vi "HFRR ADV v09.vi"() -> ()   [LabVIEW 2025] (continued)
            n2119 = Delete From Array(array=w2342, index=0) -> (array with subset deleted=w2264:dbl[])  [unwired: 1 in, 1 out]
            n2120 = Delete From Array(array=w2302, index=0) -> (array with subset deleted=w2260:dbl[])  [unwired: 1 in, 1 out]
            n2121 = Delete From Array(array=w2351, index=0) -> (array with subset deleted=w2265:dbl[])  [unwired: 1 in, 1 out]
            n2122 = Delete From Array(array=w2304, index=0) -> (array with subset deleted=w2261:dbl[])  [unwired: 1 in, 1 out]
            n2123 = Delete From Array(array=w2285, index=0) -> (array with subset deleted=w2257:dbl[])  [unwired: 1 in, 1 out]
            n2124 = Delete From Array(array=w2329, index=0) -> (array with subset deleted=w2315:dbl[])  [unwired: 1 in, 1 out]
            n2125 = Delete From Array(array=w2356, index=0) -> (array with subset deleted=w2317:dbl[])  [unwired: 1 in, 1 out]
            n2126 = Delete From Array(array=w2333, index=0) -> (array with subset deleted=w2263:dbl[])  [unwired: 1 in, 1 out]
            n2127 = Delete From Array(array=w2300, index=0) -> (array with subset deleted=w2259:dbl[])  [unwired: 1 in, 1 out]
            n2128 = Delete From Array(array=w2281, index=0) -> (array with subset deleted=w2255:dbl[])  [unwired: 1 in, 1 out]
            n2129 = Delete From Array(array=w2325, index=0) -> (array with subset deleted=w2313:dbl[])  [unwired: 1 in, 1 out]
            n2130 = Delete From Array(array=w2338, index=0) -> (array with subset deleted=w2318:dbl[])  [unwired: 1 in, 1 out]
            n2131 = Delete From Array(array=w2348, index=0) -> (array with subset deleted=w2231:dbl[])  [unwired: 1 in, 1 out]
            n2132 = Delete From Array(array=w2358, index=0) -> (array with subset deleted=w2233:dbl[])  [unwired: 1 in, 1 out]
            n2133 = Delete From Array(array=w2340, index=0) -> (array with subset deleted=w2229:dbl[])  [unwired: 1 in, 1 out]
            n2134 = Bundle "Bundle"(w2235, w2266) -> (w2253:cluster{dbl[], dbl[]})  [unwired: 1 in]
            n2135 = Bundle "Bundle"(w2235, w2320) -> (w2254:cluster{dbl[], dbl[]})  [unwired: 1 in]
            n2136 = Bundle "Bundle"(w2266, w2262) -> (w2268:cluster{dbl[], dbl[]})  [unwired: 1 in]
            n2137 = Bundle "Bundle"(w2231, w2230) -> (w2238:cluster{dbl[], dbl[]})  [unwired: 1 in]
            n2138 = Bundle "Bundle"(w2264, w2260) -> (w2270:cluster{dbl[], dbl[]})  [unwired: 1 in]
            n2139 = Bundle "Bundle"(w2231, w2264) -> (w2374:cluster{dbl[], dbl[]})  [unwired: 1 in]
            n2140 = Bundle "Bundle"(w2231, w2260) -> (w2298:cluster{dbl[], dbl[]})  [unwired: 1 in]
            n2141 = Bundle "Bundle"(w2231, w2319) -> (w2384:cluster{dbl[], dbl[]})  [unwired: 1 in]
            n2142 = Bundle "Bundle"(w2231, w2314) -> (w2322:cluster{dbl[], dbl[]})  [unwired: 1 in]
            n2143 = Bundle "Bundle"(w2231, w2345) -> (w2369:cluster{dbl[], dbl[]})  [unwired: 1 in]
            n2144 = Bundle "Bundle"(w2265, w2261) -> (w2269:cluster{dbl[], dbl[]})  [unwired: 1 in]
            n2145 = Bundle "Bundle"(w2233, w2232) -> (w2239:cluster{dbl[], dbl[]})  [unwired: 1 in]
            n2146 = Bundle "Bundle"(w2233, w2265) -> (w2376:cluster{dbl[], dbl[]})  [unwired: 1 in]
            n2147 = Bundle "Bundle"(w2233, w2261) -> (w2299:cluster{dbl[], dbl[]})  [unwired: 1 in]
            n2148 = Bundle "Bundle"(w2233, w2315) -> (w2323:cluster{dbl[], dbl[]})  [unwired: 1 in]
            n2149 = Bundle "Bundle"(w2233, w2317) -> (w2385:cluster{dbl[], dbl[]})  [unwired: 1 in]
            n2150 = Bundle "Bundle"(w2233, w2354) -> (w2367:cluster{dbl[], dbl[]})  [unwired: 1 in]
            n2151 = Bundle "Bundle"(w2263, w2259) -> (w2271:cluster{dbl[], dbl[]})  [unwired: 1 in]
            n2152 = Bundle "Bundle"(w2229, w2228) -> (w2237:cluster{dbl[], dbl[]})  [unwired: 1 in]
            n2153 = Bundle "Bundle"(w2229, w2263) -> (w2375:cluster{dbl[], dbl[]})  [unwired: 1 in]
            n2154 = Bundle "Bundle"(w2229, w2259) -> (w2297:cluster{dbl[], dbl[]})  [unwired: 1 in]
            n2155 = Bundle "Bundle"(w2229, w2313) -> (w2321:cluster{dbl[], dbl[]})  [unwired: 1 in]
            n2156 = Bundle "Bundle"(w2229, w2318) -> (w2383:cluster{dbl[], dbl[]})  [unwired: 1 in]
            n2157 = Bundle "Bundle"(w2229, w2336) -> (w2368:cluster{dbl[], dbl[]})  [unwired: 1 in]
            n2158 = call-poly <vilib>:"Mean.vi"("X"=w2316) -> ("mean"=→"CP1":dbl)  [unwired: 1 out]
            n2159 = call-poly <vilib>:"Mean.vi"("X"=w2257) -> ("mean"=→"КОФ2 3":dbl)  [unwired: 1 out]
            n2160 = call-poly <vilib>:"Mean.vi"("X"=w2315) -> ("mean"=→"CP2":dbl)  [unwired: 1 out]
            n2161 = call-poly <vilib>:"Mean.vi"("X"=w2317) -> ("mean"=→"КОФ2":dbl)  [unwired: 1 out]
            n2162 = call-poly <vilib>:"Mean.vi"("X"=w2255) -> ("mean"=→"КОФ2 5":dbl)  [unwired: 1 out]
            n2163 = call-poly <vilib>:"Mean.vi"("X"=w2313) -> ("mean"=→"CP4":dbl)  [unwired: 1 out]
            n2164 = call-poly <vilib>:"Mean.vi"("X"=w2318) -> ("mean"=→"КОФ4":dbl)  [unwired: 1 out]
            n2165 = Bundle "Bundle"(w2235, w2262) -> (w2226:cluster{dbl[], dbl[]})  [unwired: 1 in]
            n2166 = Bundle "Bundle"(w2235, w2316) -> (w2249:cluster{dbl[], dbl[]})  [unwired: 1 in]
            n2167 = Build Array "Build Array"(w2226, w2249) -> (w2252:cluster{dbl[], dbl[]}[])
            "XY Graph 17" <- w2252
            n2168 = Build Array "Build Array"(w2240, w2239, w2238, w2237) -> (→"Frequency ( Hz )":cluster{dbl[], dbl[]}[])
            n2169 = Build Array "Build Array"(w2268, w2269, w2270, w2271) -> (→"Air Temp ( °C ) vs Humidity ( % RH )":cluster{dbl[], dbl[]}[])
            n2170 = Build Array "Build Array"(w2253, w2376, w2374, w2375) -> (→"Air Temperature  ( °C )":cluster{dbl[], dbl[]}[])
            n2171 = Build Array "Build Array"(w2226, w2299, w2298, w2297) -> (→"Humidity ( %RH )":cluster{dbl[], dbl[]}[])
            n2172 = Build Array "Build Array"(w2254, w2385, w2384, w2383) -> (→"Coefficient Of Friction":cluster{dbl[], dbl[]}[])
            n2173 = Build Array "Build Array"(w2249, w2323, w2322, w2321) -> (→"Sample Temperature ( °C )":cluster{dbl[], dbl[]}[])
            n2174 = Build Array "Build Array"(w2227, w2367, w2369, w2368) -> (→"XY Graph 13":cluster{dbl[], dbl[]}[])
            n2175 = Bundle "Bundle"(w2235, w2258) -> (w2280:cluster{dbl[], dbl[]})  [unwired: 1 in]
            n2176 = Bundle "Bundle"(w2231, w2256) -> (w2278:cluster{dbl[], dbl[]})  [unwired: 1 in]
            n2177 = Bundle "Bundle"(w2233, w2257) -> (w2279:cluster{dbl[], dbl[]})  [unwired: 1 in]
            n2178 = Bundle "Bundle"(w2229, w2255) -> (w2277:cluster{dbl[], dbl[]})  [unwired: 1 in]
            n2179 = Build Array "Build Array"(w2280, w2279, w2278, w2277) -> (→"Stroke ( mm )":cluster{dbl[], dbl[]}[])
            n2180 = local write "XY Graph 16"(w2252) -> ()
          }
          frame #2 {
          }
          frame #3 {
            n2181 = local write "Numeric 8"(0 ("Numeric 8")) -> ()
            n2182 = local write "Numeric 11"(0 ("Numeric 11")) -> ()
            n2183 = local write "Numeric 12"(0 ("Numeric 12")) -> ()
            n2184 = local write "Numeric 13"(0 ("Numeric 13")) -> ()
            n2185 = property on="OPEN" class="Bool (strict)"("Visible"=TRUE) -> ()  [unwired: 2 in, 2 out]
            n2186 = local read "String Control 2"() -> (w2552:string)
            n2187 = local read "String Control 4"() -> (w2551:string)
            n2188 = local read "String Control 6"() -> (w2550:string)
            n2189 = local read "String Control 8"() -> (w2549:string)
            n2190 = Match Pattern(string=w2552, regular expression="Samples / cycle :- ") -> (after substring=w2566:string)  [unwired: 1 in, 3 out]
            n2191 = Match Pattern(string=w2552, regular expression="Frequency :- ") -> (after substring=w2585:string)  [unwired: 1 in, 3 out]
            n2192 = Match Pattern(string=w2551, regular expression="Samples / cycle :- ") -> (after substring=w2562:string)  [unwired: 1 in, 3 out]
            n2193 = Match Pattern(string=w2551, regular expression="Frequency :- ") -> (after substring=w2580:string)  [unwired: 1 in, 3 out]
            n2194 = Match Pattern(string=w2550, regular expression="Samples / cycle :- ") -> (after substring=w2558:string)  [unwired: 1 in, 3 out]
            n2195 = Match Pattern(string=w2550, regular expression="Frequency :- ") -> (after substring=w2575:string)  [unwired: 1 in, 3 out]
            n2196 = Match Pattern(string=w2549, regular expression="Samples / cycle :- ") -> (after substring=w2554:string)  [unwired: 1 in, 3 out]
            n2197 = Match Pattern(string=w2549, regular expression="Frequency :- ") -> (after substring=w2570:string)  [unwired: 1 in, 3 out]
            n2198 = String Subset(string=w2566, length (rest)=6 ("length (rest)")) -> (substring=w2568:string)  [unwired: 1 in]
            n2199 = String Subset(string=w2585, length (rest)=9 ("length (rest)")) -> (substring=w2587:string)  [unwired: 1 in]
            n2200 = String Subset(string=w2562, length (rest)=6 ("length (rest)")) -> (substring=w2564:string)  [unwired: 1 in]
            n2201 = String Subset(string=w2580, length (rest)=9 ("length (rest)")) -> (substring=w2582:string)  [unwired: 1 in]
            n2202 = String Subset(string=w2558, length (rest)=6 ("length (rest)")) -> (substring=w2560:string)  [unwired: 1 in]
            n2203 = String Subset(string=w2575, length (rest)=9 ("length (rest)")) -> (substring=w2577:string)  [unwired: 1 in]
            n2204 = String Subset(string=w2554, length (rest)=6 ("length (rest)")) -> (substring=w2556:string)  [unwired: 1 in]
            n2205 = String Subset(string=w2570, length (rest)=9 ("length (rest)")) -> (substring=w2572:string)  [unwired: 1 in]
            n2206 = Fract/Exp String To Number(string=w2568) -> (number=w2548:dbl)  [unwired: 3 in, 1 out]
            n2207 = Fract/Exp String To Number(string=w2587) -> (number=w2588:dbl)  [unwired: 3 in, 1 out]
            n2208 = Fract/Exp String To Number(string=w2564) -> (number=w2547:dbl)  [unwired: 3 in, 1 out]
            n2209 = Fract/Exp String To Number(string=w2582) -> (number=w2583:dbl)  [unwired: 3 in, 1 out]
            n2210 = Fract/Exp String To Number(string=w2560) -> (number=w2546:dbl)  [unwired: 3 in, 1 out]
            n2211 = Fract/Exp String To Number(string=w2577) -> (number=w2578:dbl)  [unwired: 3 in, 1 out]
            n2212 = Fract/Exp String To Number(string=w2556) -> (number=w2545:dbl)  [unwired: 3 in, 1 out]
            n2213 = Fract/Exp String To Number(string=w2572) -> (number=w2573:dbl)  [unwired: 3 in, 1 out]
            n2214 = local write "sample1"(w2548) -> ()
            n2215 = local write "freq1"(w2588) -> ()
            n2216 = local write "sample2"(w2547) -> ()
            n2217 = local write "freq2"(w2583) -> ()
            n2218 = local write "sample3"(w2546) -> ()
            n2219 = local write "freq3"(w2578) -> ()
            n2220 = local write "sample4"(w2545) -> ()
            n2221 = local write "freq 4"(w2573) -> ()
          }
        }
      }
    }
    n2222 = case shown="True" w2035 {
      selector: w2035 -> [_ w2164]
      frame False {
      }
      frame True {
        n2223 = Not(x=w2164) -> (.not. x?=w2160:bool)
        n2224 = local write "service 3"(w2160) -> ()
        n2225 = local write "OPEN 6"(w2160) -> ()
        n2226 = call <vilib>:"System Exec.vi"("wait until completion? (T)"=TRUE, "command line"="C:\\LAB-IQ\\Scar View.exe") -> ("error out"=→"error out 5":errorcluster)  [unwired: 6 in, 3 out]
      }
    }
    n2227 = case shown="\"Acquire\", Default" w2047 {
      frame "Acquire", Default {
        w3084 = 0.2 ("y")
        w3089 = 1.0 ("y")
        w3090 = 0.8 ("y")
        # "Elapsed time\ncof\nstroke\nAir temp\nTemp\nHumidity"
        n2228 = disable-structure shown="Disabled" {
          frame Disabled {
            n2229 = local read "Flag"() -> (w3107:dbl)
            n2230 = local read "RUN"() -> (w3104:bool)
            n2231 = Not(x=w3104) -> (.not. x?=w3103:bool)
            n2232 = Equal?(x=w3107, y=10.0) -> (x = y?=w3105:bool)
            n2233 = And(x=w3105, y=w3103) -> (x .and. y?=w3102:bool)
            n2234 = case shown="True" w3102 {
              frame False {
              }
              frame True {
                w3108 = FALSE ("Heater Button")
                n2235 = local write "Humidity"(w3108) -> ()
                n2236 = local write "Heater Button"(w3108) -> ()
              }
            }
          }
          frame Enabled {
          }
        }
        n2237 = disable-structure shown="Disabled" {
          frame Disabled {
            n2238 = case shown="True" {
              selector: _ -> [_ _]
              frame False {
              }
              frame True {
                w3199 = TRUE ("Heater")
                n2239 = local write "Humidity"(w3199) -> ()
                n2240 = local write "Heater Button"(w3199) -> ()
                n2241 = local read "TEST STANDARD"() -> (w3202:T3)
                n2242 = local read "TEST STANDARD"() -> (w3197:T3)
                n2243 = Equal?(x=w3202, y=enum16{"ASTM D6079", "ISO 12156", "Custom"}."ISO 12156" ("Test Standard")) -> (x = y?=w3200:bool)
                n2244 = Equal?(x=w3197, y=enum16{"ASTM D6079", "ISO 12156", "Custom"}."ASTM D6079" ("Test Standard")) -> (x = y?=w3196:bool)
                n2245 = case shown="True" w3200 {
                  frame False {
                  }
                  frame True {
                    n2246 = local write "Heater"(TRUE ("Heater")) -> ()
                    n2247 = local write "airtempflg"(FALSE ("airtempflg")) -> ()
                  }
                }
                n2248 = case shown="True" w3196 {
                  frame False {
                  }
                  frame True {
                    n2249 = local write "Heater"(FALSE ("Heater")) -> ()
                    n2250 = local write "airtempflg"(TRUE ("airtempflg")) -> ()
                  }
                }
              }
            }
          }
          frame Enabled {
          }
        }
        n2251 = stacked-sequence {
          frame #0 {
            n2252 = case shown="True" "RST FF" {
              frame False {
              }
              frame True {
                w3265 = 0.0 ("X Scale.Range:Maximum")
                n2253 = property on="Frictional Force ( N )" class="WFChart (strict)"("XScale.Maximum"=600.0 ("X Scale.Range:Maximum"), "XScale.Minimum"=w3265, "YScale.Maximum"=10.0 ("Y Scale.Range:Maximum"), "YScale.Minimum"=w3265) -> ()  [unwired: 2 in, 2 out]
              }
            }
          }
          frame #1 {
            n2254 = case shown="True" "RST TEMP" {
              frame False {
              }
              frame True {
                n2255 = property on="Temperature ( Deg C )" class="WFChart (strict)"("XScale.Minimum"=0.0 ("X Scale.Range:Minimum"), "XScale.Maximum"=600.0 ("X Scale.Range:Maximum"), "YScale.Minimum"=0.0 ("Y Scale.Range:Minimum"), "YScale.Maximum"=100.0 ("Y Scale.Range:Maximum")) -> ()  [unwired: 2 in, 2 out]
              }
            }
          }
          frame #2 {
            n2256 = case shown="True" "RSTCOF" {
              frame False {
              }
              frame True {
                n2257 = property on="Coefficient of Friction" class="WFChart (strict)"("XScale.Minimum"=0.0 ("X Scale.Range:Minimum"), "XScale.Maximum"=600.0 ("X Scale.Range:Maximum"), "YScale.Maximum"=1.0 ("X Scale.Range:Minimum"), "YScale.Minimum"=0.0 ("X Scale.Range:Minimum")) -> ()  [unwired: 2 in, 2 out]
              }
            }
          }
          frame #3 {
            n2258 = case shown="True" "RSTCOF 2" {
              frame False {
              }
              frame True {
                (unwired) 100.0 ("Y Scale.Range:Maximum")
                (unwired) 0.0 ("Y Scale.Range:Minimum")
                (unwired) 600.0 ("X Scale.Range:Maximum")
                (unwired) 0.0 ("X Scale.Range:Minimum")
              }
            }
          }
          frame #4 {
            n2259 = case shown="True" "RSTCOF 3" {
              frame False {
              }
              frame True {
                n2260 = property on="Electrical Contact Resistance ( % )" class="WFChart (strict)"("XScale.Minimum"=0.0 ("X Scale.Range:Minimum"), "XScale.Maximum"=600.0 ("X Scale.Range:Maximum"), "YScale.Minimum"=0.0 ("Y Scale.Range:Minimum"), "YScale.Maximum"=100.0 ("Y Scale.Range:Maximum")) -> ()  [unwired: 2 in, 2 out]
              }
            }
          }
        }
        n2261 = disable-structure shown="Disabled" {
          frame Disabled {
            n2262 = case shown="True" {
              selector: _ -> [_ _]
              frame False {
              }
              frame True {
                n2263 = local read "zflag 2"() -> (w3166:dbl)
                n2264 = local read "yflag"() -> (w3168:dbl)
                n2265 = Equal?(x=w3168, y=2.0 ("tflag")) -> (x = y?=w3170:bool)
                n2266 = Equal?(x=w3166, y=3.0 ("tflag")) -> (x = y?=w3169:bool)
                n2267 = And(x=w3170, y=w3169) -> (x .and. y?=w3164:bool)
                n2268 = case shown="True" w3164 {
                  frame False {
                  }
                  frame True {
                    w3195 = 0.0 ("zflag")
                    n2269 = local write "zflag"(w3195) -> ()
                    n2270 = local write "zflag 2"(w3195) -> ()
                    n2271 = Delete(path (use dialog)=path "C:/LAB-IQ-NXT/WO 2449 TT.sig" ("file path (dialog if empty)")) -> (deleted path=w3194:path)  [unwired: 4 in, 2 out]
                    n2272 = Delete(path (use dialog)=path "C:/LAB-IQ-NXT/WO 2449 TRH.sig" ("file path (dialog if empty)")) -> (deleted path=w3189:path)  [unwired: 4 in, 2 out]
                    n2273 = local read "SEN.RUN HRS"() -> (w3181:dbl)
                    n2274 = local read "SENSOR TIME"() -> (w3179:dbl)
                    n2275 = call <vilib>:"compatOverwrite.vi"("overwrite (F)"=TRUE) -> ("overwrite?"=w3171:T25)
                    n2276 = call <vilib>:"compatOverwrite.vi"("overwrite (F)"=TRUE) -> ("overwrite?"=w3175:T25)
                    n2277 = local read "Total No. of Tests"() -> (w3182:dbl)
                    n2278 = Add(x=w3179, y=w3181) -> (x+y=w3180:dbl)
                    "SEN.RUN HRS" <- w3180
                    n2279 = Open/Create/Replace File(file path (use dialog)=w3194, operation (0:open)=w3171) -> (refnum out=w3172:refnum<file>, error out=w3173:errorcluster)  [unwired: 4 in, 1 out]
                    n2280 = Open/Create/Replace File(file path (use dialog)=w3189, operation (0:open)=w3175) -> (refnum out=w3176:refnum<file>, error out=w3177:errorcluster)  [unwired: 4 in, 1 out]
                    n2281 = Deny Access(4:w3173, 6:T23."deny none" ("deny mode (2)"), 7:w3172) -> (3:w3193:refnum<file>)  [unwired: 1 out]
                    n2282 = Deny Access(4:w3177, 6:T23."deny none" ("deny mode (2)"), 7:w3176) -> (3:w3185:refnum<file>)  [unwired: 1 out]
                    n2283 = Number To Decimal String(number=w3182) -> (decimal integer string=w3190:string)  [unwired: 1 in]
                    n2284 = Number To Decimal String(number=w3180) -> (decimal integer string=w3186:string)  [unwired: 1 in]
                    n2285 = Write to Binary File(file (use dialog)=w3193, data=w3190, 5:FALSE ("prepend array or string size? (T)")) -> ()  [unwired: 3 in, 3 out]
                    n2286 = Write to Binary File(file (use dialog)=w3185, data=w3186, 5:FALSE ("prepend array or string size? (T)")) -> ()  [unwired: 3 in, 3 out]
                  }
                }
              }
            }
          }
          frame Enabled {
          }
        }
        n2287 = local read "RUN"() -> (w3093:bool)
        n2288 = local read "run replace"() -> (w3097:bool)
        n2289 = local read "run replace"() -> (w3096:bool)
        n2290 = case shown="True" w3093 {
          frame False {
            n2291 = local write "run replace"(FALSE ("run replace")) -> ()
          }
          frame True {
            "run replace" <- TRUE ("run replace")
          }
        }
        n2292 = local read "RUN"() -> (w3101:bool)
        n2293 = local read "Set Temp"() -> (w3063:dbl)
        n2294 = local read "SetTemp"() -> (w3065:dbl)
        n2295 = case shown="False" w3101 {
          tunnel: [FALSE ("TEST RUNNING") TRUE ("TEST RUNNING")] -> w3100
          frame False {
            w3284 = 0.0 ("Flag")
            n2296 = local write "Elapsed time"(0.0 ("elapsedtime")) -> ()
            n2297 = local write "Time Remaining"(w3284) -> ()
            n2298 = local write "Flag"(w3284) -> ()
            n2299 = local write "Remaining Time"(w3284) -> ()
          }
          frame True {
            n2300 = local write "Flag"(10.0 ("Flag")) -> ()
          }
        }
        n2301 = case shown="False" w3097 {
          frame False {
            n2302 = local read "zflag"() -> (→"zflag 2":dbl)
            n2303 = local write "yflag"(2.0 ("tflag")) -> ()
            n2304 = local write "FLAG 4"(0.0 ("FLAG")) -> ()
          }
          frame True {
            n2305 = local write "yflag"(1.0 ("tflag")) -> ()
            n2306 = local write "zflag"(3.0 ("zflag")) -> ()
          }
        }
        n2307 = local read "acq 2"() -> (w3095:bool)
        n2308 = local read "AIR TEMP"() -> (w3058:dbl)
        n2309 = local read "Amb temp"() -> (w3062:dbl)
        n2310 = case shown="True" "Save & Continue" {
          frame False {
          }
          frame True {
            "acq 2" <- TRUE ("acq 2")
          }
        }
        n2311 = local read "Set Rh"() -> (w3064:dbl)
        n2312 = Add(x=w3065, y=w3090) -> (x+y=w3091:dbl)
        n2313 = Subtract(x=w3065, y=w3090) -> (x-y=w3092:dbl)
        n2314 = Add(x=w3063, y=w3084) -> (x+y=w3085:dbl)
        n2315 = Subtract(x=w3063, y=w3084) -> (x-y=w3086:dbl)
        n2316 = And(x=w3095, y=w3096) -> (x .and. y?=w3094:bool)
        n2317 = Greater Or Equal?(x=w3058, y=15.0) -> (x >= y?=w3059:bool)
        "powstat" <- w3059
        n2318 = local read "Humidity ( %RH )"() -> (w3061:dbl)
        n2319 = case shown="True" "Save & Continue" {
          frame False {
          }
          frame True {
            n2320 = while {
              tunnel: "0123456789abcdefghijklmnopqrstuvwxyzABCDEFGHIJKLMNOPQRSTUVWXYZ" ("string 2") -> [w3255]
              shift-right: [w3253] -> w3248
              shift-left: "" -> [w3252]
              i -> [w3262]
              stop <- w3261 stop-if-true
              n2321 = Random Number (0-1)() -> (number: 0 to 1=w3256:dbl)
              n2322 = Multiply(x=w3256, y=62.0) -> (x*y=w3258:dbl)
              n2323 = Decrement(x="Length") -> (x-1=w3251:i16)
              n2324 = To Word Integer(number=w3258) -> (16bit integer=w3259:i16)
              n2325 = String Subset(string=w3255, offset (0)=w3259, length (rest)=1 ("length (rest)")) -> (substring=w3254:string)
              n2326 = Greater Or Equal?(x=w3262, y=w3251) -> (x >= y?=w3261:bool)
              n2327 = Concatenate Strings(w3254, w3252) -> (w3253:string)
            }
            n2328 = local write "UUID"(w3248) -> ()
          }
        }
        n2329 = In Range and Coerce(upper limit=w3091, x=w3062, lower limit=w3092) -> (In Range?=w3081:bool)  [unwired: 1 out]
        n2330 = Add(x=w3064, y=w3089) -> (x+y=w3088:dbl)
        n2331 = Subtract(x=w3064, y=w3089) -> (x-y=w3087:dbl)
        n2332 = local read "TEMP"() -> (w3060:dbl)
        n2333 = case shown="True" "Save & Continue" {
          frame False {
          }
          frame True {
            n2334 = local read "Operator ID"() -> (w3604:string)
            n2335 = local read "FILE"() -> (w3610:string)
            n2336 = String Length(string=w3610) -> (length=w3608:i32)
            n2337 = String Length(string=w3604) -> (length=w3605:i32)
            n2338 = Greater?(x=w3608, y=0) -> (0:w3607:bool)
            n2339 = Greater?(x=w3605, y=0) -> (0:w3603:bool)
            n2340 = And(x=w3607, y=w3603) -> (x .and. y?=w3602:bool)
            n2341 = case shown="True" w3602 {
              frame False {
                n2342 = stacked-sequence {
                  frame #0 {
                    n2343 = One Button Dialog(message="Please Enter a File Name and Operator ID to save data !", button name ("OK")="Ok") -> ()  [unwired: 1 out]
                  }
                  frame #1 {
                    n2344 = local write "Save & Continue"(FALSE ("OK Button")) -> ()
                  }
                }
                n2345 = local write "Save & Continue"(FALSE ("OK Button")) -> ()
              }
              frame True {
                n2346 = stacked-sequence {
                  frame #0 {
                    n2347 = local read "FILE"() -> (w3616:string)
                    n2348 = call "file check.vi"("file name in"=w3616) -> ("file name out"=w3615:string)  [unwired: 9 in, 1 out]
                    n2349 = call <vilib>:"Application Directory.vi"() -> ("Application Directory"=w3626:path)
                    n2350 = Build Path(base path=w3626, name or relative path="data") -> (appended path=w3625:path)
                    n2351 = call <vilib>:"Trim Whitespace.vi"("string"=w3615) -> ("trimmed string"=w3623:string)  [unwired: 1 in]
                    n2352 = call <vilib>:"Trim Whitespace.vi"("string"=w3615) -> ("trimmed string"=w3624:string)  [unwired: 1 in]
                    n2353 = List Folder(path=w3625) -> (folder names=w3621:string[])  [unwired: 3 in, 3 out]
                    n2354 = Match Pattern(string=w3623, regular expression="_(") -> (before substring=w3620:string)  [unwired: 1 in, 3 out]
                    n2355 = for {
                      tunnel: w3621 -> [w3635] mode=indexing
                      tunnel: w3620 -> [w3633]
                      shift-right: [w3631] -> w3618
                      shift-left: bool[] [] -> [w3632]
                      n2356 = Match Pattern(string=w3635, regular expression="_(") -> (before substring=w3634:string)  [unwired: 1 in, 3 out]
                      n2357 = Equal?(x=w3634, y=w3633) -> (x = y?=w3630:bool)
                      n2358 = case shown="True" w3630 {
                        tunnel: w3630 -> [_ w3638]
                        tunnel: w3632 -> [w3637 w3640]
                        tunnel: [w3637 w3639] -> w3631
                        frame False {
                        }
                        frame True {
                          n2359 = Insert Into Array(array=w3640, new element=w3638) -> (w3639:bool[])  [unwired: 1 in]
                        }
                      }
                    }
                    n2360 = Equal?(x=w3621, y=w3620) -> (x = y?=w3629:bool[])
                    n2361 = Or Array Elements(Boolean array=w3629) -> (logical OR=w3628:bool)
                    n2362 = Array Size(array=w3618) -> (size(s)=w3617:i32)
                    n2363 = case shown="True" w3628 {
                      tunnel: w3624 -> [_ w3648]
                      tunnel: w3617 -> [_ w3641]
                      frame False {
                      }
                      frame True {
                        n2364 = Number To Decimal String(number=w3641) -> (decimal integer string=w3644:string)  [unwired: 1 in]
                        n2365 = Search/Split String(string=w3648, search string/char (-)="_(" ("regular expression")) -> (substring before match=w3646:string)  [unwired: 1 in, 2 out]
                        n2366 = Concatenate Strings(w3646, "_(" ("regular expression"), w3644, ")" ("regular expression")) -> (w3642:string)
                        n2367 = local write "FILE"(w3642) -> ()
                      }
                    }
                  }
                  frame #1 {
                    w3649 = 0.0
                    w3662 = cluster{"y":dbl, dbl, "y":dbl}[] [] ("History Data")
                    w3663 = FALSE ("Heater Button")
                    (unwired) ")!" ("string")
                    (unwired) ")" ("string")
                    w3661 = dbl[] [] ("History Data")
                    w3667 = "\r"
                    # "C:\\WinDucom\\Data\\"
                    # "C:\\LAB-IQ-NXT\\data"
                    n2368 = local write "Humidity ( %RH )"(w3649) -> ()
                    n2369 = local write "Frequency ( Hz )"(w3649) -> ()
                    n2370 = local write "Stroke 3"(w3649) -> ()
                    n2371 = local write "speedop"(0.0 ("PIDclk 2")) -> ()
                    n2372 = local write "Set Temp 2"(65.0 ("Set Temp 2")) -> ()
                    n2373 = local write "AIR TEMP"(w3649) -> ()
                    n2374 = local write "clk"(0.0 ("clk")) -> ()
                    n2375 = local write "Stroke 4"(w3649) -> ()
                    n2376 = local write "Stroke"(w3649) -> ()
                    n2377 = local write "COF 3"(w3649) -> ()
                    n2378 = local write "COF 2"(w3649) -> ()
                    n2379 = local write "TEMP"(w3649) -> ()
                    n2380 = local write "ecr 3"(w3649) -> ()
                    n2381 = local write "FF 3"(w3649) -> ()
                    n2382 = local write "FF 2"(w3649) -> ()
                    n2383 = property on="Humidity ( %RH )" class="WFChart (strict)"("History Data"=w3661) -> ()  [unwired: 2 in, 2 out]
                    n2384 = property on="Coefficient of Friction" class="WFChart (strict)"("History Data"=w3661) -> ()  [unwired: 2 in, 2 out]
                    n2385 = property on="Coefficient of Friction" class="WFChart (strict)"("History Data"=w3661) -> ()  [unwired: 2 in, 2 out]
                    n2386 = property on="Frictional Force ( N )" class="WFChart (strict)"("History Data"=w3661) -> ()  [unwired: 2 in, 2 out]
                    n2387 = property on="Electrical Contact Resistance ( % )" class="WFChart (strict)"("History Data"=w3661) -> ()  [unwired: 2 in, 2 out]
                    n2388 = property on="Electrical Contact Resistance ( % )" class="WFChart (strict)"("History Data"=w3661) -> ()  [unwired: 2 in, 2 out]
                    n2389 = property on="Temperature ( Deg C )" class="WFChart (strict)"("History Data"=w3661) -> ()  [unwired: 2 in, 2 out]
                    n2390 = property on="Frictional Force ( N )" class="WFChart (strict)"("History Data"=w3661) -> ()  [unwired: 2 in, 2 out]
                    n2391 = property on="Coefficient of Friction" class="WFChart (strict)"("History Data"=w3661) -> ()  [unwired: 2 in, 2 out]
                    n2392 = property on="Frictional Force ( N )" class="WFChart (strict)"("History Data"=w3661) -> ()  [unwired: 2 in, 2 out]
                    n2393 = property on="Electrical Contact Resistance ( % )" class="WFChart (strict)"("History Data"=w3661) -> ()  [unwired: 2 in, 2 out]
                    n2394 = property on="Temperature ( Deg C )" class="WFChart (strict)"("History Data"=w3661) -> ()  [unwired: 2 in, 2 out]
                    n2395 = property on="Humidity ( %RH )" class="WFChart (strict)"("History Data"=w3661) -> ()  [unwired: 2 in, 2 out]
                    n2396 = property on="Stroke ( mm )" class="WFChart (strict)"("History Data"=w3662) -> ()  [unwired: 2 in, 2 out]
                    n2397 = property on="Stroke ( mm )" class="WFChart (strict)"("History Data"=w3662) -> ()  [unwired: 2 in, 2 out]
                    n2398 = local write "Humidity"(w3663) -> ()
                    n2399 = local write "Heater Button"(w3663) -> ()
                    n2400 = local read "FILE"() -> (w3657:string)
                    n2401 = local read "NORMAL LOAD"() -> (w3682:dbl)
                    n2402 = call "file check.vi"("file name in"=w3657) -> ("error out"=w3660:errorcluster, "file name out"=w3654:string)  [unwired: 9 in]
                    n2403 = call "FILE PATH CREATION.vi"("error in"=w3660, "FILE NAME :"=w3654) -> ("FILE OUT"=w3653:path)  [unwired: 8 in, 1 out]
                    n2404 = Concatenate Strings(w3654, ".dgf" ("Substring")) -> (w3659:string)
                    n2405 = Concatenate Strings(w3654, ".duf" ("Substring")) -> (w3655:string)
                    n2406 = Multiply(x=w3682, y=1.0) -> (x*y=w3681:dbl)
                    n2407 = Build Path(base path=w3653, name or relative path=w3659) -> (appended path=w3652:path)
                    n2408 = Build Path(base path=w3653, name or relative path=w3655) -> (appended path=w3651:path)
                    n2409 = Number To Fractional String(number=w3681, width (-)=i16 5, precision (6)=i16 2) -> (F-format string=w3690:string)  [unwired: 1 in]
                    n2410 = local read "Fuel Discription :"() -> (w3677:string)
                    n2411 = local read "Batch Ref Num :"() -> (w3665:string)
                    n2412 = Get Date/Time String(date format (0)=enum16{"short", "long", "abbreviated"}."short") -> (date string=w3701:string, time string=w3698:string)  [unwired: 2 in]
                    n2413 = local read "Remarks :"() -> (w3676:string)
                    n2414 = Concatenate Strings("Load :- " ("Substring"), w3690, " N ," ("Substring")) -> (w3689:string)
                    n2415 = local read "String 41"() -> (w3668:string)
                    n2416 = Concatenate Strings(w3677) -> (w3678:string)
                    n2417 = Concatenate Strings(w3665) -> (w3664:string)
                    n2418 = Concatenate Strings("tested by") -> (w3672:string)
                    n2419 = Concatenate Strings("(" ("Substring"), w3701, ")" ("Substring"), w3698) -> (w3670:string)
                    "concatenated string" <- w3670
                    n2420 = Concatenate Strings(w3676, "," ("string")) -> (w3675:string)
                    n2421 = Concatenate Strings("  TIME;      COF;       STROKE;     AIR TEMP;  TEMP;  HUMIDITY;  ECR; PID-OUT; FREQUENCY" ("Substring"), "\r") -> (w3685:string)
                    n2422 = Concatenate Strings(w3668, w3667, "Fuel Discription :-" ("Substring"), w3678, w3667, w3689, w3667, "Batch Ref Num :-" ("Substring"), w3664, w3667, " Remarks :- " ("Substring"), w3675, w3667, " Date :- " ("Substring"), w3670, w3667, "Tested By :-" ("Substring"), w3672) -> (w3683:string)
                    "REMARKS" <- w3683
                    n2423 = call <vilib>:"Write Characters To File.vi"("append to file? (new file:F)"=FALSE, "character string"=w3685, "file path (dialog if empty)"=w3652) -> ()  [unwired: 2 in, 1 out]
                    n2424 = call <vilib>:"Write Characters To File.vi"("append to file? (new file:F)"=FALSE, "character string"=w3683, "file path (dialog if empty)"=w3651) -> ()  [unwired: 2 in, 1 out]
                  }
                  frame #2 {
                    n2425 = local write "Cycles elapsed"(0 ("Cycles elapsed")) -> ()
                    n2426 = local write "cyclecount"(0 ("cyclecount")) -> ()
                    n2427 = local write "Save & Continue"(FALSE ("OK")) -> ()
                    n2428 = local write "autostrtflg"(TRUE ("autostrtflg")) -> ()
                    n2429 = local write "Save"(FALSE ("Save")) -> ()
                    n2430 = Get Date/Time In Seconds() -> (seconds since 1Jan1904=w3707:timestamp)
                    n2431 = To Double Precision Float(number=w3707) -> (double precision float=w3706:dbl)
                    n2432 = local write "acq timer"(w3706) -> ()
                    n2433 = One Button Dialog(message="Please ensure sample is mounted properly and machine is ready in all aspects for testing !", button name ("OK")="Ok") -> ()  [unwired: 1 out]
                  }
                  frame #3 {
                    n2434 = stacked-sequence {
                      frame #0 {
                        n2435 = local write "Main Dashboard Buttons"(T1."Dashboard" ("Main Dashboard Buttons")) -> ()
                        n2436 = local write "Main Tab"(T2."Acquire" ("Main Tab")) -> ()
                      }
                      frame #1 {
                        n2437 = local write "EVENT LOG"("" ("EVENT LOG")) -> ()
                      }
                      frame #2 {
                        n2438 = Wait (ms)(milliseconds to wait=u32 50) -> ()  [unwired: 1 out]
                      }
                      frame #3 {
                        n2439 = disable-structure shown="Disabled" {
                          frame Disabled {
                            n2440 = local read "EVENT LOG"() -> (w3719:string)
                            n2441 = call "Event Log.vi"("Content"="Test Details", "EVENT LOG"=w3719) -> ("EVENT LOG"=w3718:string)  [unwired: 8 in, 1 out]
                            n2442 = local write "EVENT LOG"(w3718) -> ()
                          }
                          frame Enabled {
                          }
                        }
                      }
                      frame #4 {
                        n2443 = Wait (ms)(milliseconds to wait=u32 50) -> ()  [unwired: 1 out]
                      }
                      frame #5 {
                        n2444 = local read "FILE"() -> (w3721:string)
                        n2445 = Concatenate Strings("File Name :" ("Content"), w3721) -> (w3722:string)
                        n2446 = local read "EVENT LOG"() -> (w3725:string)
                        n2447 = call "Event Log.vi"("Content"=w3722, "EVENT LOG"=w3725) -> ("EVENT LOG"=w3724:string)  [unwired: 8 in, 1 out]
                        n2448 = local write "EVENT LOG"(w3724) -> ()
                      }
                      frame #6 {
                        n2449 = Wait (ms)(milliseconds to wait=u32 50) -> ()  [unwired: 1 out]
                      }
                      frame #7 {
                        n2450 = local read "Batch Ref Num :"() -> (w3727:string)
                        n2451 = Concatenate Strings("Batch Ref No :" ("Content"), w3727) -> (w3728:string)
                        n2452 = local read "EVENT LOG"() -> (w3731:string)
                        n2453 = call "Event Log.vi"("Content"=w3728, "EVENT LOG"=w3731) -> ("EVENT LOG"=w3730:string)  [unwired: 8 in, 1 out]
                        n2454 = local write "EVENT LOG"(w3730) -> ()
                      }
                      frame #8 {
                        n2455 = Wait (ms)(milliseconds to wait=u32 50) -> ()  [unwired: 1 out]
                      }
                      frame #9 {
                        n2456 = local read "tested by"() -> (w3733:string)
                        n2457 = Concatenate Strings("Tested By :" ("Content"), w3733) -> (w3734:string)
                        n2458 = local read "EVENT LOG"() -> (w3737:string)
                        n2459 = call "Event Log.vi"("Content"=w3734, "EVENT LOG"=w3737) -> ("EVENT LOG"=w3736:string)  [unwired: 8 in, 1 out]
                        n2460 = local write "EVENT LOG"(w3736) -> ()
                      }
                      frame #10 {
                        n2461 = Wait (ms)(milliseconds to wait=u32 50) -> ()  [unwired: 1 out]
                      }
                      frame #11 {
                        n2462 = local read "TEST STANDARD"() -> (w3740:T3)
                        n2463 = case shown="\"ASTM D6079\", Default" w3740 {
                          tunnel: ["ASTM D6079" "ISO 12156" "CEC F-096-A-06" "Custom"] -> w3739
                          frame "ASTM D6079", Default {
                          }
                          frame "ISO 12156" {
                          }
                          frame "CEC F-096-A-06" {
                          }
                          frame "Custom" {
                          }
                        }
                        n2464 = Concatenate Strings("Test Standard :" ("Content"), w3739) -> (w3741:string)
                        n2465 = local read "EVENT LOG"() -> (w3744:string)
                        n2466 = call "Event Log.vi"("Content"=w3741, "EVENT LOG"=w3744) -> ("EVENT LOG"=w3743:string)  [unwired: 8 in, 1 out]
                        n2467 = local write "EVENT LOG"(w3743) -> ()
                      }
                      frame #12 {
                        n2468 = Wait (ms)(milliseconds to wait=u32 50) -> ()  [unwired: 1 out]
                      }
                      frame #13 {
                        n2469 = local read "Fuel Discription :"() -> (w3750:string)
                        n2470 = Concatenate Strings("Fuel Description :" ("Content"), w3750) -> (w3751:string)
                        n2471 = local read "EVENT LOG"() -> (w3754:string)
                        n2472 = call "Event Log.vi"("Content"=w3751, "EVENT LOG"=w3754) -> ("EVENT LOG"=w3753:string)  [unwired: 8 in, 1 out]
                        n2473 = local write "EVENT LOG"(w3753) -> ()
                      }
                      frame #14 {
                        n2474 = Wait (ms)(milliseconds to wait=u32 50) -> ()  [unwired: 1 out]
                      }
                      frame #15 {
                        n2475 = local read "Remarks :"() -> (w3756:string)
                        n2476 = Concatenate Strings("Remarks :" ("Content"), w3756) -> (w3757:string)
                        n2477 = local read "EVENT LOG"() -> (w3760:string)
                        n2478 = call "Event Log.vi"("Content"=w3757, "EVENT LOG"=w3760) -> ("EVENT LOG"=w3759:string)  [unwired: 8 in, 1 out]
                        n2479 = local write "EVENT LOG"(w3759) -> ()
                      }
                      frame #16 {
                        n2480 = Wait (ms)(milliseconds to wait=u32 50) -> ()  [unwired: 1 out]
                      }
                      frame #17 {
                        n2481 = local read "Operator ID"() -> (w3762:string)
                        n2482 = Concatenate Strings("Operator ID :" ("Content"), w3762) -> (w3764:string)
                        n2483 = local read "EVENT LOG"() -> (w3766:string)
                        n2484 = call "Event Log.vi"("Content"=w3764, "EVENT LOG"=w3766) -> ("EVENT LOG"=w3765:string)  [unwired: 8 in, 1 out]
                        n2485 = local write "EVENT LOG"(w3765) -> ()
                      }
                      frame #18 {
                        n2486 = Wait (ms)(milliseconds to wait=u32 50) -> ()  [unwired: 1 out]
                      }
                      frame #19 {
                        n2487 = disable-structure shown="Disabled" {
                          frame Disabled {
                            n2488 = local read "EVENT LOG"() -> (w3770:string)
                            n2489 = call "Event Log.vi"("Content"="Test Parameter", "EVENT LOG"=w3770) -> ("EVENT LOG"=w3769:string)  [unwired: 8 in, 1 out]
                            n2490 = local write "EVENT LOG"(w3769) -> ()
                          }
                          frame Enabled {
                          }
                        }
                      }
                      frame #20 {
                        n2491 = Wait (ms)(milliseconds to wait=u32 50) -> ()  [unwired: 1 out]
                      }
                      frame #21 {
                        n2492 = local read "Set Hz"() -> (w3774:dbl)
                        n2493 = Number To Fractional String(number=w3774, precision (6)=i16 2) -> (F-format string=w3773:string)  [unwired: 2 in]
                        n2494 = Concatenate Strings("Set Frequency [Hz] :" ("Content"), w3773) -> (w3776:string)
                        n2495 = local read "EVENT LOG"() -> (w3778:string)
                        n2496 = call "Event Log.vi"("Content"=w3776, "EVENT LOG"=w3778) -> ("EVENT LOG"=w3777:string)  [unwired: 8 in, 1 out]
                        n2497 = local write "EVENT LOG"(w3777) -> ()
                      }
                      frame #22 {
                        n2498 = Wait (ms)(milliseconds to wait=u32 50) -> ()  [unwired: 1 out]
                      }
                      frame #23 {
                        n2499 = local read "NORMAL LOAD"() -> (w3781:dbl)
                        n2500 = Number To Fractional String(number=w3781, precision (6)=i16 2) -> (F-format string=w3782:string)  [unwired: 2 in]
                        n2501 = Concatenate Strings("Applied Load [N] :" ("Content"), w3782) -> (w3784:string)
                        n2502 = local read "EVENT LOG"() -> (w3786:string)
                        n2503 = call "Event Log.vi"("Content"=w3784, "EVENT LOG"=w3786) -> ("EVENT LOG"=w3785:string)  [unwired: 8 in, 1 out]
                        n2504 = local write "EVENT LOG"(w3785) -> ()
                      }
                      frame #24 {
                        n2505 = Wait (ms)(milliseconds to wait=u32 50) -> ()  [unwired: 1 out]
                      }
                      frame #25 {
                        n2506 = local read "Set Strk"() -> (w3789:dbl)
                        n2507 = Number To Fractional String(number=w3789, precision (6)=i16 2) -> (F-format string=w3790:string)  [unwired: 2 in]
                        n2508 = Concatenate Strings("Set Stroke [mm] :" ("Content"), w3790) -> (w3792:string)
                        n2509 = local read "EVENT LOG"() -> (w3794:string)
                        n2510 = call "Event Log.vi"("Content"=w3792, "EVENT LOG"=w3794) -> ("EVENT LOG"=w3793:string)  [unwired: 8 in, 1 out]
                        n2511 = local write "EVENT LOG"(w3793) -> ()
                      }
                      frame #26 {
                        n2512 = Wait (ms)(milliseconds to wait=u32 50) -> ()  [unwired: 1 out]
                      }
                      frame #27 {
                        n2513 = local read "Set Temp"() -> (w3797:dbl)
                        n2514 = Number To Fractional String(number=w3797, precision (6)=i16 2) -> (F-format string=w3798:string)  [unwired: 2 in]
                        n2515 = Concatenate Strings("Set Temperature [deg C] :" ("Content"), w3798) -> (w3800:string)
                        n2516 = local read "EVENT LOG"() -> (w3802:string)
                        n2517 = call "Event Log.vi"("Content"=w3800, "EVENT LOG"=w3802) -> ("EVENT LOG"=w3801:string)  [unwired: 8 in, 1 out]
                        n2518 = local write "EVENT LOG"(w3801) -> ()
                      }
                      frame #28 {
                        n2519 = Wait (ms)(milliseconds to wait=u32 50) -> ()  [unwired: 1 out]
                      }
                      frame #29 {
                        n2520 = local read "Set Rh"() -> (w3805:dbl)
                        n2521 = Number To Fractional String(number=w3805, precision (6)=i16 2) -> (F-format string=w3806:string)  [unwired: 2 in]
                        n2522 = Concatenate Strings("Set Humidity [%RH] :" ("Content"), w3806) -> (w3808:string)
                        n2523 = local read "EVENT LOG"() -> (w3810:string)
                        n2524 = call "Event Log.vi"("Content"=w3808, "EVENT LOG"=w3810) -> ("EVENT LOG"=w3809:string)  [unwired: 8 in, 1 out]
                        n2525 = local write "EVENT LOG"(w3809) -> ()
                      }
                      frame #30 {
                        n2526 = Wait (ms)(milliseconds to wait=u32 50) -> ()  [unwired: 1 out]
                      }
                      frame #31 {
                        n2527 = local read "test time"() -> (w3813:dbl)
                        n2528 = Number To Fractional String(number=w3813, precision (6)=i16 1) -> (F-format string=w3814:string)  [unwired: 2 in]
                        n2529 = Concatenate Strings("Test Duration [mins] :" ("Content"), w3814) -> (w3816:string)
                        n2530 = local read "EVENT LOG"() -> (w3818:string)
                        n2531 = call "Event Log.vi"("Content"=w3816, "EVENT LOG"=w3818) -> ("EVENT LOG"=w3817:string)  [unwired: 8 in, 1 out]
                        n2532 = local write "EVENT LOG"(w3817) -> ()
                      }
                      frame #32 {
                        w3819 = dbl[] [] ("History Data")
                        w3820 = cluster{"y":dbl, dbl, "y":dbl}[] [] ("History Data")
                        w3821 = FALSE ("Visible")
                        n2533 = property on="Stroke ( mm )" class="WFChart (strict)"("History Data"=w3820) -> ()  [unwired: 2 in, 2 out]
                        n2534 = property on="Humidity ( %RH )" class="WFChart (strict)"("History Data"=w3819) -> ()  [unwired: 2 in, 2 out]
                        n2535 = property on="Temperature ( Deg C )" class="WFChart (strict)"("History Data"=w3819) -> ()  [unwired: 2 in, 2 out]
                        n2536 = property on="Electrical Contact Resistance ( % )" class="WFChart (strict)"("History Data"=w3819) -> ()  [unwired: 2 in, 2 out]
                        n2537 = property on="Coefficient of Friction" class="WFChart (strict)"("History Data"=w3819) -> ()  [unwired: 2 in, 2 out]
                        n2538 = property on="Frictional Force ( N )" class="WFChart (strict)"("History Data"=w3819) -> ()  [unwired: 2 in, 2 out]
                        n2539 = property on="Coefficient of Friction" class="WFChart (strict)"("History Data"=w3819) -> ()  [unwired: 2 in, 2 out]
                        n2540 = property on="Frictional Force ( N )" class="WFChart (strict)"("History Data"=w3819) -> ()  [unwired: 2 in, 2 out]
                        n2541 = property on="Electrical Contact Resistance ( % )" class="WFChart (strict)"("History Data"=w3819) -> ()  [unwired: 2 in, 2 out]
                        n2542 = property on="Humidity ( %RH )" class="WFChart (strict)"("History Data"=w3819) -> ()  [unwired: 2 in, 2 out]
                        n2543 = property on="Stroke ( mm )" class="WFChart (strict)"("History Data"=w3820) -> ()  [unwired: 2 in, 2 out]
                        n2544 = property on="Temperature ( Deg C )" class="WFChart (strict)"("History Data"=w3819) -> ()  [unwired: 2 in, 2 out]
                        n2545 = property on="Service Password Log" class="Str"("Visible"=w3821) -> ()  [unwired: 2 in, 2 out]
                        n2546 = property on="Password 3" class="Clust (strict)"("Visible"=w3821) -> ()  [unwired: 2 in, 2 out]
                      }
                    }
                    "TEST FILE NAM,E SAVED" <- TRUE ("TEST FILE NAM,E SAVED")
                  }
                }
              }
            }
          }
        }
        n2547 = case shown="True" w3094 {
          frame False {
            n2548 = local write "tfalg"(0.0 ("tfalg")) -> ()
          }
          frame True {
            n2549 = local read "tfalg"() -> (w3239:dbl)
            n2550 = Equal?(x=w3239, y=0.0) -> (x = y?=w3240:bool)
            n2551 = case shown="True" w3240 {
              frame False {
              }
              frame True {
                n2552 = local read "Total No. of Tests"() -> (w3243:dbl)
                n2553 = local write "tfalg"(1.0 ("tfalg")) -> ()
                n2554 = local write "acq 2"(FALSE ("acq 2")) -> ()
                n2555 = Wait (ms)(milliseconds to wait=u32 200) -> ()  [unwired: 1 out]
                n2556 = Increment(x=w3243) -> (x+1=w3242:dbl)
                n2557 = local write "Total No. of Tests"(w3242) -> ()
              }
            }
          }
        }
        n2558 = local write "Test \nStatus"(w3100) -> ()
        n2559 = local write "st enable"(w3100) -> ()
        n2560 = local write "PWR"(w3100) -> ()
        n2561 = local write "Save"(w3100) -> ()
        n2562 = local read "Main Tab"() -> (w3057:T2)
        n2563 = case shown="True" w3081 {
          tunnel: [FALSE ("RUN") TRUE ("RUN")] -> w3080
          tunnel: [_ 1] -> w3073
          frame False {
          }
          frame True {
          }
        }
        n2564 = In Range and Coerce(upper limit=w3088, x=w3061, lower limit=w3087) -> (In Range?=w3079:bool)  [unwired: 1 out]
        n2565 = In Range and Coerce(upper limit=w3085, x=w3060, lower limit=w3086) -> (In Range?=w3077:bool)  [unwired: 1 out]
        n2566 = case shown="True" w3093 {
          frame False {
            n2567 = local read "Rt 3"() -> (w3221:bool)
            n2568 = case shown="True" w3221 {
              frame False {
              }
              frame True {
                n2569 = local write "Rt 3"(FALSE ("Rt 3")) -> ()
                n2570 = local write "Json End Flg"(TRUE ("Upld AR 2")) -> ()
              }
            }
            "Rt" <- TRUE ("Rt")
            "Rt 2" <- FALSE ("Rt")
          }
          frame True {
            n2571 = local read "Rt"() -> (w3228:bool)
            n2572 = local write "Rt 2"(TRUE ("Rt 2")) -> ()
            n2573 = case shown="True" w3228 {
              frame False {
              }
              frame True {
                w3229 = TRUE ("Upld AR 2")
                n2574 = local write "Rt"(FALSE ("Rt")) -> ()
                n2575 = local write "Upld AR"(w3229) -> ()
                n2576 = local write "Json St Flg"(w3229) -> ()
              }
            }
            "Rt 3" <- TRUE ("Rt 3")
          }
        }
        n2577 = case shown="True" w3079 {
          tunnel: [FALSE ("RUN") TRUE ("RUN")] -> w3078
          tunnel: [_ 2] -> w3072
          frame False {
          }
          frame True {
          }
        }
        n2578 = case shown="True" w3077 {
          tunnel: [FALSE ("RUN") TRUE ("RUN")] -> w3076
          tunnel: [_ 3] -> w3071
          frame False {
          }
          frame True {
          }
        }
        n2579 = case shown="\"Acquire\"" w3057 {
          tunnel: w3059 -> [_ w3290]
          frame Default {
            w3289 = 0.0 ("output")
            n2580 = local write "PID-out"(w3289) -> ()
            n2581 = local write "Frequency ( Hz )"(w3289) -> ()
          }
          frame "Acquire" {
            n2582 = stacked-sequence {
              frame #0 {
                n2583 = local read "Auto Start Test"() -> (w3292:bool)
                n2584 = case shown="True" w3292 {
                  tunnel: "RUN" -> [w3313 w3316]
                  tunnel: [w3313 w3315] -> w3293
                  frame False {
                  }
                  frame True {
                    n2585 = local read "Auto Start Temp"() -> (w3314:bool)
                    n2586 = Or(x=w3316, y=w3314) -> (x .or. y?=w3315:bool)
                  }
                }
                n2587 = local read "clk"() -> (w3312:dbl)
                n2588 = local read "Save"() -> (w3308:bool)
                n2589 = Equal?(x=w3312, y=0.0) -> (x = y?=w3309:bool)
                n2590 = And(x=w3309, y=w3308) -> (x .and. y?=w3310:bool)
                n2591 = Not(x="Engage") -> (.not. x?=w3299:bool)
                n2592 = case shown="True" w3293 {
                  tunnel: [w3324 w3342] -> w3295
                  frame False {
                    w3324 = 0.0
                    n2593 = local read "Auto Start Test"() -> (w3320:bool)
                    n2594 = local write "Reinit PID"(TRUE) -> ()
                    n2595 = local write "Start Time"(TRUE ("Start Time")) -> ()
                    n2596 = property on="Stroke" class="DigNum (strict)"("Visible"=TRUE) -> ()  [unwired: 2 in, 2 out]
                    n2597 = property on="Stroke 2" class="DigNum (strict)"("Visible"=FALSE) -> ()  [unwired: 2 in, 2 out]
                    n2598 = case shown="False" w3320 {
                      frame False {
                        n2599 = property on="Heater Button" class="Bool (strict)"("DisabledEnum"=T15."Enabled" ("Disabled")) -> ()  [unwired: 2 in, 2 out]
                        n2600 = property on="Humidity" class="Bool (strict)"("DisabledEnum"=T15."Enabled" ("Disabled")) -> ()  [unwired: 2 in, 2 out]
                      }
                      frame True {
                      }
                    }
                    n2601 = case shown="False" "TestCompFlg" {
                      frame False {
                        n2602 = local read "StartFlg"() -> (w3330:bool)
                        n2603 = case shown="True" w3330 {
                          frame False {
                          }
                          frame True {
                            n2604 = flat-sequence {
                              frame #0 {
                                n2605 = local read "EVENT LOG"() -> (w3332:string)
                                n2606 = call "Event Log.vi"("Content"="Test was interrupted", "EVENT LOG"=w3332) -> ("EVENT LOG"=w3333:string)  [unwired: 8 in, 1 out]
                                n2607 = local write "EVENT LOG"(w3333) -> ()
                              }
                              frame #1 {
                                w3334 = FALSE ("StartFlg")
                                n2608 = local write "Heater Button"(w3334) -> ()
                                n2609 = local write "StartFlg"(w3334) -> ()
                                n2610 = local write "Humidity"(w3334) -> ()
                              }
                            }
                          }
                        }
                      }
                      frame True {
                      }
                    }
                    n2611 = local write "String 14"("Test will autostart once parameters reach the set value." ("String 14")) -> ()
                    n2612 = local write "Old Pid Val"(w3324) -> ()
                  }
                  frame True {
                    n2613 = property on="Stroke 2" class="DigNum (strict)"("Visible"=TRUE) -> ()  [unwired: 2 in, 2 out]
                    n2614 = property on="Stroke" class="DigNum (strict)"("Visible"=FALSE) -> ()  [unwired: 2 in, 2 out]
                    n2615 = property on="STOP 2" class="Bool (strict)"("Disabled"=u8 2) -> ()  [unwired: 2 in, 2 out]
                    n2616 = local write "String 14"(" Running....." ("String 14")) -> ()
                    n2617 = property on="Heater Button" class="Bool (strict)"("DisabledEnum"=T15."Disabled and Grayed Out" ("Disabled")) -> ()  [unwired: 2 in, 2 out]
                    n2618 = property on="Humidity" class="Bool (strict)"("DisabledEnum"=T15."Disabled and Grayed Out" ("Disabled")) -> ()  [unwired: 2 in, 2 out]
                    n2619 = local read "PID Ref"() -> (w3353:bool)
                    n2620 = case shown="True" w3353 {
                      tunnel: [w3359 w3375] -> w3352
                      frame False {
                        n2621 = local read "Old Pid Val"() -> (w3359:dbl)
                      }
                      frame True {
                        n2622 = local read "Set Hz"() -> (w3368:dbl)
                        n2623 = local read "Frequency"() -> (w3379:dbl)
                        n2624 = Add(x=w3368, y=10.0) -> (x+y=w3377:dbl)
                        n2625 = Add(x=w3368, y=-10.0 ("Offset")) -> (x+y=w3386:dbl)
                        n2626 = Add(x=w3368, y=-10.0) -> (x+y=w3378:dbl)
                        n2627 = In Range and Coerce(upper limit=w3377, x=w3379, lower limit=w3378) -> (coerced(x)=w3367:dbl)  [unwired: 1 out]
                        n2628 = Or(x="Reinit PID", y="Reinit PID") -> (x .or. y?=w3376:bool)
                        n2629 = Multiply(x=w3386, y=0.1 ("Gain")) -> (x*y=w3365:dbl)
                        n2630 = local read "Elapsed time"() -> (w3372:dbl)
                        n2631 = local read "SPEED OUT:"() -> (w3387:dbl)
                        n2632 = Add(x=w3365, y=1.5) -> (x+y=w3363:dbl)
                        n2633 = call-poly <vilib>:"PID.vi"("reinitialize? (F)"=w3376, "output range"=cluster{"output high":dbl, "output low":dbl} {"output high"=1.0, "output low"=-1.0}, "PID gains"=T12 {"proportional gain (Kc)"=0.0005, "integral time (Ti, min)"=0.001, "derivative time (Td, min)"=0.0} ("Motor PID"), "process variable"=w3367, "setpoint"=w3368) -> ("output"=w3366:dbl)  [unwired: 5 in, 1 out]
                        n2634 = Multiply(x=w3363, y=w3387) -> (x*y=w3362:dbl)
                        n2635 = Greater?(x=w3372, y=0.05) -> (0:w3371:bool)
                        n2636 = case shown="True" w3371 {
                          tunnel: w3366 -> [_ w3389]
                          tunnel: [0.0 ("output") w3389] -> w3369
                          frame False {
                          }
                          frame True {
                            n2637 = local write "Reinit PID"(FALSE ("Reinit PID")) -> ()
                          }
                        }
                        n2638 = Multiply(x=w3362, y=0.8) -> (x*y=w3361:dbl)
                        n2639 = Add(x=w3361, y=w3369) -> (x+y=w3374:dbl)
                        n2640 = flat-sequence {
                          tunnel: [w3392] -> w3375
                          tunnel: w3374 -> [w3392]
                          frame #0 {
                            n2641 = local write "PID Ref"(FALSE ("PID Ref")) -> ()
                          }
                        }
                      }
                    }
                    "Old Pid Val" <- w3352
                    n2642 = case shown="True" "Start Time" {
                      selector: "Start Time" -> [_ w3355]
                      frame False {
                      }
                      frame True {
                        n2643 = Not(x=w3355) -> (.not. x?=w3354:bool)
                        n2644 = local write "Start Time"(w3354) -> ()
                        n2645 = local read "EVENT LOG"() -> (w3356:string)
                        n2646 = call "Event Log.vi"("Content"="Test in progress", "EVENT LOG"=w3356) -> ("EVENT LOG"=w3358:string)  [unwired: 8 in, 1 out]
                        n2647 = local write "EVENT LOG"(w3358) -> ()
                      }
                    }
                    n2648 = local read "Set Hz"() -> (w3349:dbl)
                    n2649 = call <vilib>:"Uniform White Noise Waveform.vi"() -> ("signal out"=w3348:waveform(dbl))  [unwired: 10 in, 1 out]
                    n2650 = local read "Freq"() -> (w3341:dbl)
                    n2651 = Add(x=w3349, y=w3348) -> (x+y=w3347:waveform(dbl))
                    n2652 = Multiply(x=w3347, y=ext 0.1) -> (x*y=w3343:waveform(ext))
                    n2653 = Multiply(x=w3341, y=0.9) -> (x*y=w3344:dbl)
                    n2654 = Add(x=w3343, y=w3344) -> (x+y=w3342:waveform(ext))
                    "StartFlg" <- TRUE ("StartFlg")
                  }
                }
                n2655 = case shown="True" w3310 {
                  frame False {
                  }
                  frame True {
                    n2656 = local write "clk"(10.0 ("clk")) -> ()
